vi "get_HS_version.vi"(8 "error in (no error)":errorcluster, 9 "string in":string) -> (0 "error out":errorcluster, 1 "version number edited string out":string, 2 "version number out":string)   [LabVIEW 2010, in "ErrorController.lvclass"]
uses:
  ErrorController.lvclass
  tools/HelioUpdateMH100803/HelioUpdateMH100803/HelioUpdateMH100803.lvclass
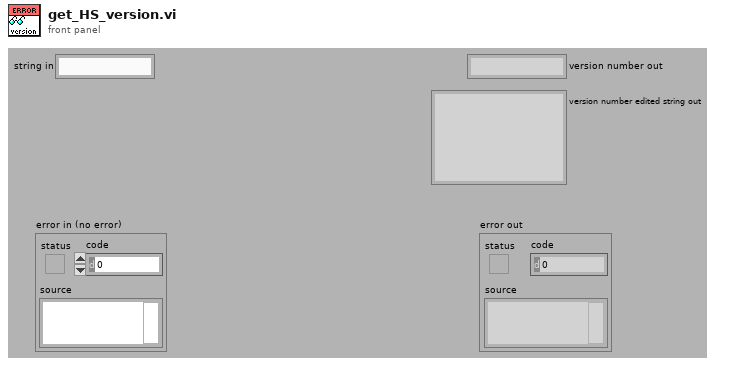
[diagram p1: front panel]
types:
  T1 = enum16{"open", "replace", "create", "open or create", "replace or create", "replace or create with confirmation"}
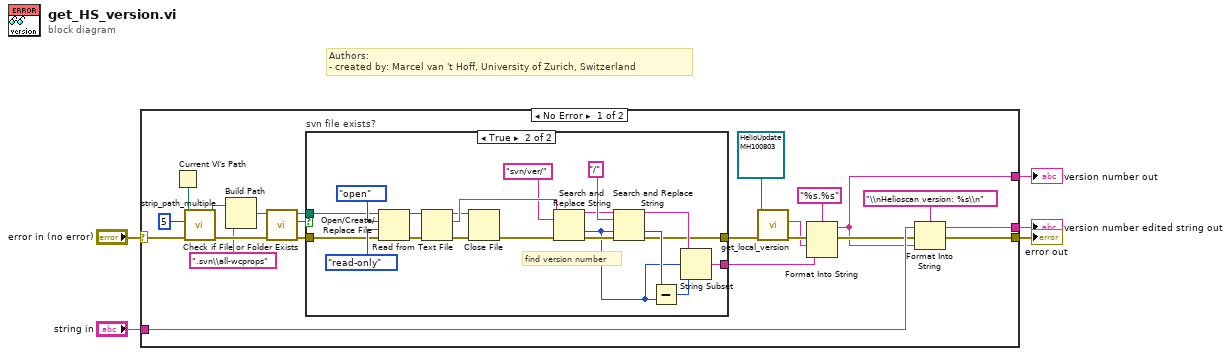
[diagram p0: block diagram]
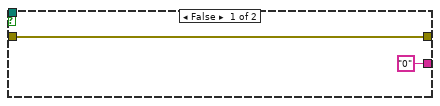
[diagram p2: hidden frame]
diagram:
  # "Authors: \n- created by: Marcel van 't Hoff, University of Zurich, Switzerland"
  n1 = case shown="No Error" "error in (no error)" {
    selector: "error in (no error)" -> [w13 w50]
    tunnel: [w26 w50] -> w4
    tunnel: [w16 _] -> w3
    tunnel: [w27 _] -> w2
    tunnel: "string in" -> [w24 _]
    frame No Error {
      n2 = Current VI's Path() -> (path=w15:path)
      n3 = call "strip_path_multiple.vi"("error in (no error)"=w13, "number of strips"=5, "path in"=w15) -> ("error out"=w9:errorcluster, "path out"=w10:path)  [unwired: 7 in]
      n4 = Build Path(base path=w10, name or relative path=".svn\\all-wcprops") -> (appended path=w8:path)
      n5 = call <vilib>:"Check if File or Folder Exists.vi"("error in (no error)"=w9, "path"=w8) -> ("error out"=w11:errorcluster, "file or folder exists?"=w12:bool, "dup path"=w6:path)  [unwired: 7 in]
      n6 = case "svn file exists?" shown="True" w12 {
        tunnel: w11 -> [w29 w30]
        tunnel: [w29 w33] -> w22
        tunnel: ["0" ("result string") w32] -> w18
        tunnel: w6 -> [_ w31]
        frame False {
        }
        frame True {
          # "find version number"
          n7 = Open/Create/Replace File(file path (use dialog)=w31, error in=w30, operation (0:open)=T1."open", access (0:read/write)=enum16{"read/write", "read-only", "write-only"}."read-only") -> (refnum out=w36:refnum<file>, error out=w37:errorcluster)  [unwired: 2 in, 1 out]
          n8 = Read from Text File(file (use dialog)=w36, error in=w37) -> (refnum out=w38:refnum<file>, text=w45:string, error out=w39:errorcluster)  [unwired: 2 in, 1 out]
          n9 = Close File(refnum=w38, error in=w39) -> (error out=w48:errorcluster)  [unwired: 1 out]
          n10 = Search and Replace String(input string=w45, search string="svn/ver/", error in=w48) -> (result string=w41:string, offset past replacement=w43:i32, error out=w49:errorcluster)  [unwired: 5 in, 1 out]
          n11 = Search and Replace String(input string=w41, search string="/", offset=w43, error in=w49) -> (result string=w46:string, offset past replacement=w47:i32, error out=w33:errorcluster)  [unwired: 4 in, 1 out]
          n12 = Subtract(x=w47, y=w43) -> (x-y=w44:i32)
          n13 = String Subset(string=w46, offset (0)=w43, length (rest)=w44) -> (substring=w32:string)
        }
      }
      n14 = call-dynamic "get_local_version.vi"("error in (no error)"=w22, "HelioUpdateMH100803 in"=refnum<class "HelioUpdateMH100803.lvclass"> refnum) -> ("error out"=w21:errorcluster, "local version out"=w19:string)  [unwired: 6 in, 2 out]
      n15 = Format Into String(format string="%s.%s", error in=w21, w19, w18) -> (resulting string=w16:string, error out=w20:errorcluster)  [unwired: 1 in]
      n16 = Format Into String(format string="\\nHelioscan version: %s\\n", initial string=w24, error in=w20, w16) -> (resulting string=w27:string, error out=w26:errorcluster)
    }
    frame Error {
    }
  }
  "error out" <- w4
  "version number out" <- w3
  "version number edited string out" <- w2
